vi "Numeros Randomicos.vi"() -> ()   [LabVIEW 2020]
panel:
  out "i":i32
  out "numero generado":dbl
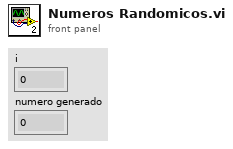
[diagram p1: front panel]
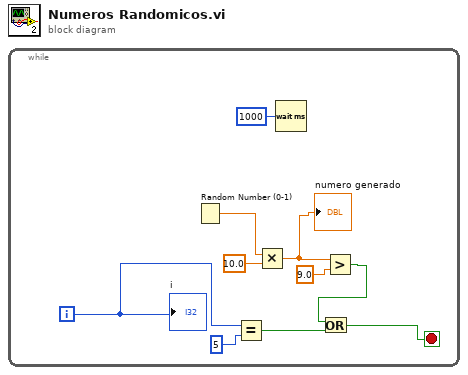
[diagram p0: block diagram]
diagram:
  n1 = while {
    i -> [w3]
    stop <- w4 stop-if-true
    n2 = Random Number (0-1)() -> (number: 0 to 1=w10:dbl)
    n3 = Equal?(x=w3, y=5 ("x")) -> (x = y?=w1:bool)
    n4 = Multiply(x=w10, y=10.0) -> (x*y=w8:dbl)
    "numero generado" <- w8
    n5 = Wait (ms)(milliseconds to wait=u32 1000) -> ()  [unwired: 1 out]
    n6 = Greater?(x=w8, y=9.0 ("x")) -> (0:w5:bool)
    n7 = Or(x=w5, y=w1) -> (x .or. y?=w4:bool)
    "i" <- w3
  }
